vi "Align Mask and Signal - wfm.vi"(4 "Mask Selector":u16(ring) items=["ITU", "EIA/TIA 547-1989"], 6 "trigger index":i32, 8 "error in (no error)":errorcluster, 9 "lower limit":waveform(dbl), 10 "upper limit":waveform(dbl), 11 "Waveform":waveform(dbl)={"t0"=timestamp(0 s since 1904-01-01), "dt"=0.0, "Y"=[]}) -> (0 "error out":errorcluster, 1 "lower limit out":waveform(dbl), 2 "upper limit out":waveform(dbl), 3 "Waveform out":waveform(dbl), 5 "Subset Waveform":waveform(dbl))   [LabVIEW 2018]
doc: "The pulse mask tests sampled data corresponding to a quarter cycle before the trigger point. With a sampling period of 10 ns, 16 samples correspond to a quarter cycle."
uses:
  <vilib>/Waveform/WDTOps.llb/WDT Number of Waveform Samples DBL.vi
  <vilib>/Waveform/WDTOps.llb/WDT Get Waveform Subset DBL (LV80).vi
  <vilib>/Waveform/WDTOps.llb/WDT Align Waveform Timestamps DBL.vi
  <vilib>/Analysis/NI_AALBase.lvlib
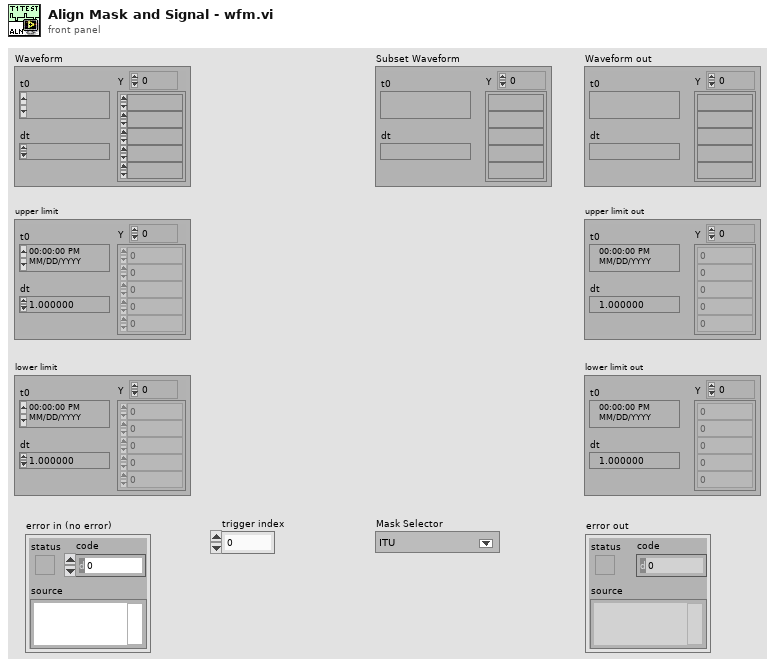
[diagram p1: front panel]
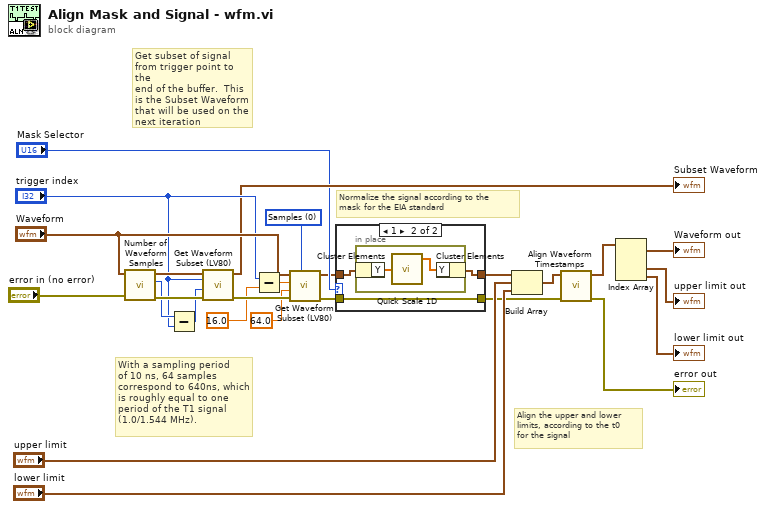
[diagram p0: block diagram]
diagram:
  w1 = u16 0 items=["Samples", "Absolute Time", "Relative Time"] ("start/duration format")
  # "Normalize the signal according to the \nmask for the EIA standard"
  # "Align the upper and lower\nlimits, according to the t0 \nfor the signal"
  # "With a sampling period\nof 10 ns, 64 samples\ncorrespond to 640ns, which\nis roughly equal to one\nperiod of the T1 signal\n(1.0/1.544 MHz)."
  # "Get subset of signal\nfrom trigger point to the\nend of the buffer.  This\nis the Subset Waveform\nthat will be used on the \nnext iteration"
  n1 = call-poly <vilib>:"Number of Waveform Samples.vi"("error in (no error)"="error in (no error)", "waveform in"="Waveform") -> ("error out"=w16:errorcluster, "number of samples"=w14:i32, "waveform out"=w17:waveform(dbl))  [unwired: 7 in]
  n2 = Subtract(x=w14, y="trigger index") -> (x-y=w12:i32)
  n3 = call-poly <vilib>:"Get Waveform Subset (LV80).vi"("error in (no error)"=w16, "duration"=w12, "start samples/time"="trigger index", "waveform in"=w17) -> ("error out"=w15:errorcluster, "waveform out"=→"Subset Waveform":waveform(dbl))  [unwired: 2 in, 2 out]
  n4 = Subtract(x="trigger index", y=16.0) -> (x-y=w18:dbl)
  n5 = call-poly <vilib>:"Get Waveform Subset (LV80).vi"("start/duration format"=w1, "error in (no error)"=w15, "duration"=64.0, "start samples/time"=w18, "waveform in"="Waveform") -> ("error out"=w9:errorcluster, "waveform out"=w7:waveform(dbl))  [unwired: 1 in, 2 out]
  n6 = case shown="1" "Mask Selector" {
    tunnel: w9 -> [w28 w31]
    tunnel: [w28 w31] -> w8
    tunnel: w7 -> [w27 w30]
    tunnel: [w27 w29] -> w6
    frame 0, Default {
    }
    frame 1 {
      n7 = in-place {
        n8 = in-place-cluster #1(w30) -> ("Y"=w32:dbl[])
        n9 = call <vilib>:"Quick Scale 1D.vi"("X"=w32) -> ("Y[i]=X[i]/Max|X|"=w33:dbl[])  [unwired: 2 out]
        n10 = in-place-cluster #1("Y"=w33) -> (w29:waveform(dbl))
      }
    }
  }
  n11 = Build Array(w6, "upper limit", "lower limit") -> (w22:waveform(dbl)[])
  n12 = call-poly <vilib>:"Align Waveform Timestamps.vi"("error in (no error)"=w8, "waveforms in"=w22) -> ("error out"=→"error out":errorcluster, "waveforms out"=w21:waveform(dbl)[])  [unwired: 8 in]
  n13 = Index Array(array=w21) -> (element #1=→"Waveform out":waveform(dbl), element #2=→"upper limit out":waveform(dbl), element #3=→"lower limit out":waveform(dbl))  [unwired: 3 in]
